vi "All Comd.vi"(7 "指令":cluster{"指令":string, "是否运行":bool}[](array[cluster]), 8 "error in":errorcluster, 11 "queue in":T1) -> (0 "error out":errorcluster, 3 "queue out":T1)   [LabVIEW 2011]
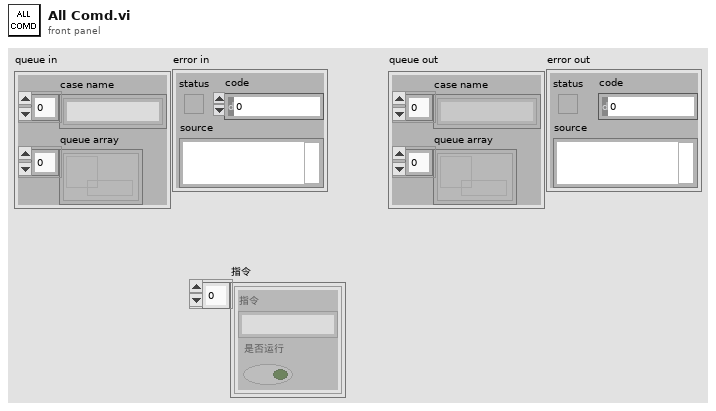
[diagram p1: front panel]
types:
  T1 = cluster{"case name":string[], "queue array":refnum<queue>[]}
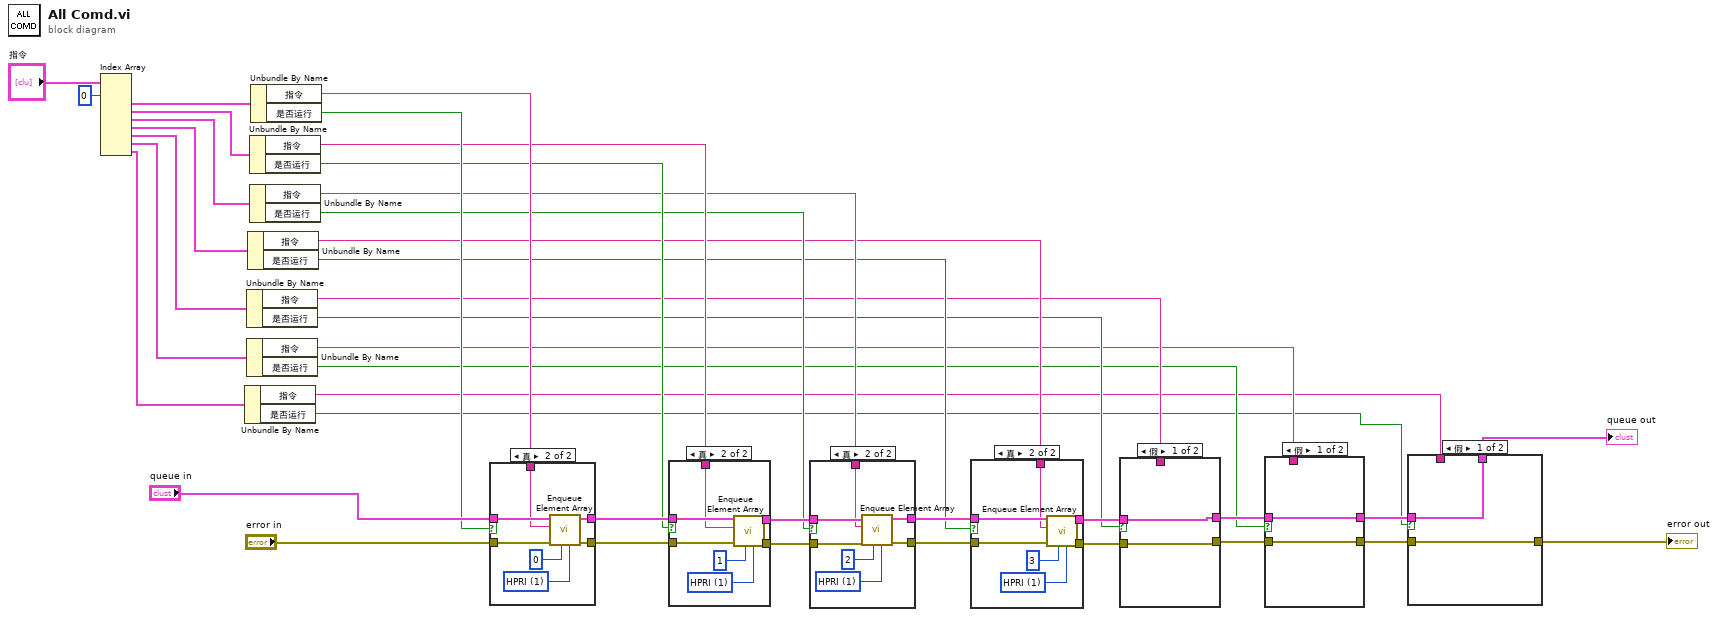
[diagram p0: block diagram]
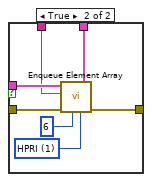
[diagram p2: hidden frame]
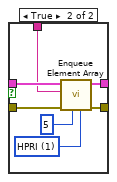
[diagram p3: hidden frame]
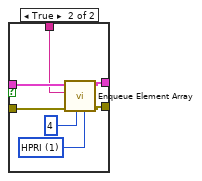
[diagram p4: hidden frame]
diagram:
  n1 = Index Array(array="指令", index #1=0 ("索引")) -> (element #1=w21:cluster{"指令":string, "是否运行":bool}, element #3=w18:cluster{"指令":string, "是否运行":bool}, element #4=w17:cluster{"指令":string, "是否运行":bool}, element #5=w16:cluster{"指令":string, "是否运行":bool}, element #6=w15:cluster{"指令":string, "是否运行":bool}, element #7=w14:cluster{"指令":string, "是否运行":bool}, element #8=w13:cluster{"指令":string, "是否运行":bool})  [unwired: 7 in, 1 out]
  n2 = Unbundle By Name(w13) -> ("指令"=w2:string, "是否运行"=w1:bool)
  n3 = Unbundle By Name(w15) -> ("指令"=w6:string, "是否运行"=w5:bool)
  n4 = Unbundle By Name(w14) -> ("指令"=w4:string, "是否运行"=w3:bool)
  n5 = Unbundle By Name(w16) -> ("指令"=w8:string, "是否运行"=w7:bool)
  n6 = Unbundle By Name(w18) -> ("指令"=w12:string, "是否运行"=w11:bool)
  n7 = Unbundle By Name(w17) -> ("指令"=w10:string, "是否运行"=w9:bool)
  n8 = Unbundle By Name(w21) -> ("指令"=w20:string, "是否运行"=w19:bool)
  n9 = case shown="真" w19 {
    tunnel: [w41 w46] -> w39
    tunnel: [w40 w45] -> w36
    tunnel: "queue in" -> [w41 w44]
    tunnel: "error in" -> [w40 w43]
    tunnel: w20 -> [_ w42]
    frame False {
    }
    frame True {
      w48 = u16 1 items=["HPRI"=1, "LPRI"=0] ("priority")
      n10 = call "Enqueue Element Array.vi"("priority"=w48, "queue index"=0, "error in"=w43, "master data"=w42, "queue in"=w44) -> ("error out"=w45:errorcluster, "queue out"=w46:T1)  [unwired: 5 in]
    }
  }
  n11 = case shown="真" w11 {
    tunnel: w39 -> [w50 w55]
    tunnel: [w50 w54] -> w38
    tunnel: w36 -> [w49 w53]
    tunnel: [w49 w52] -> w35
    tunnel: w12 -> [_ w51]
    frame False {
    }
    frame True {
      w56 = u16 1 items=["HPRI"=1, "LPRI"=0] ("priority")
      n12 = call "Enqueue Element Array.vi"("priority"=w56, "queue index"=1, "error in"=w53, "master data"=w51, "queue in"=w55) -> ("error out"=w52:errorcluster, "queue out"=w54:T1)  [unwired: 5 in]
    }
  }
  n13 = case shown="真" w9 {
    tunnel: w38 -> [w59 w64]
    tunnel: [w59 w63] -> w37
    tunnel: w35 -> [w58 w62]
    tunnel: [w58 w61] -> w34
    tunnel: w10 -> [_ w60]
    frame False {
    }
    frame True {
      w66 = u16 1 items=["HPRI"=1, "LPRI"=0] ("priority")
      n14 = call "Enqueue Element Array.vi"("priority"=w66, "queue index"=2, "error in"=w62, "master data"=w60, "queue in"=w64) -> ("error out"=w61:errorcluster, "queue out"=w63:T1)  [unwired: 5 in]
    }
  }
  n15 = case shown="真" w7 {
    tunnel: w37 -> [w68 w73]
    tunnel: w34 -> [w67 w72]
    tunnel: [w68 w71] -> w33
    tunnel: [w67 w70] -> w32
    tunnel: w8 -> [_ w69]
    frame False {
    }
    frame True {
      w74 = u16 1 items=["HPRI"=1, "LPRI"=0] ("priority")
      n16 = call "Enqueue Element Array.vi"("priority"=w74, "queue index"=3, "error in"=w72, "master data"=w69, "queue in"=w73) -> ("error out"=w70:errorcluster, "queue out"=w71:T1)  [unwired: 5 in]
    }
  }
  n17 = case shown="假" w5 {
    tunnel: w33 -> [w77 w82]
    tunnel: w32 -> [w76 w81]
    tunnel: [w77 w80] -> w31
    tunnel: [w76 w79] -> w30
    tunnel: w6 -> [_ w78]
    frame False {
    }
    frame True {
      w84 = u16 1 items=["HPRI"=1, "LPRI"=0] ("priority")
      n18 = call "Enqueue Element Array.vi"("priority"=w84, "queue index"=4, "error in"=w81, "master data"=w78, "queue in"=w82) -> ("error out"=w79:errorcluster, "queue out"=w80:T1)  [unwired: 5 in]
    }
  }
  n19 = case shown="假" w3 {
    tunnel: w31 -> [w86 w91]
    tunnel: w30 -> [w85 w90]
    tunnel: [w86 w89] -> w29
    tunnel: [w85 w88] -> w28
    tunnel: w4 -> [_ w87]
    frame False {
    }
    frame True {
      w92 = u16 1 items=["HPRI"=1, "LPRI"=0] ("priority")
      n20 = call "Enqueue Element Array.vi"("priority"=w92, "queue index"=5, "error in"=w90, "master data"=w87, "queue in"=w91) -> ("error out"=w88:errorcluster, "queue out"=w89:T1)  [unwired: 5 in]
    }
  }
  n21 = case shown="假" w1 {
    tunnel: w29 -> [w94 w100]
    tunnel: w28 -> [w95 w99]
    tunnel: [w94 w98] -> w26
    tunnel: [w95 w97] -> w25
    tunnel: w2 -> [_ w96]
    frame False {
    }
    frame True {
      w102 = u16 1 items=["HPRI"=1, "LPRI"=0] ("priority")
      n22 = call "Enqueue Element Array.vi"("priority"=w102, "queue index"=6, "error in"=w99, "master data"=w96, "queue in"=w100) -> ("error out"=w97:errorcluster, "queue out"=w98:T1)  [unwired: 5 in]
    }
  }
  "queue out" <- w26
  "error out" <- w25
